vi "LabVIEW_Set Temperature.vi"(0 "PC Comms Port":refnum<visa-resource-name>="COM3", 5 "Air Temperature Setpoint (°C)":dbl=37.5 min=25.0 max=80.0 step=0.1, 11 "error in (no error)":errorcluster) -> (4 "PC Comms Port Out":refnum<visa-resource-name>="COM3", 15 "error out":errorcluster)   [LabVIEW 2010]
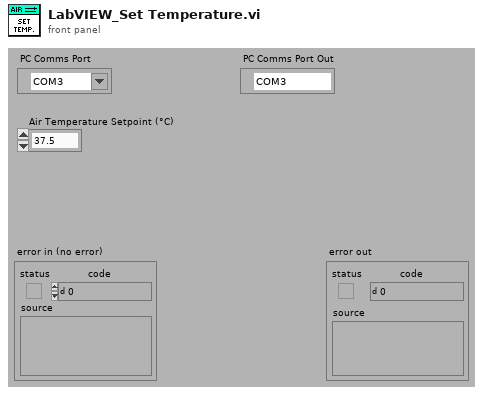
[diagram p1: front panel]
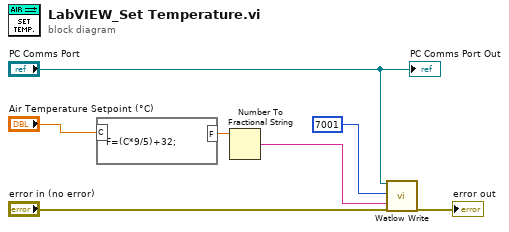
[diagram p0: block diagram]
diagram:
  n1 = formula code="F=(C*9/5)+32;"("C"="Air Temperature Setpoint (°C)") -> ("F"=w6:dbl)
  n2 = Number To Fractional String(number=w6) -> (F-format string=w5:string)  [unwired: 3 in]
  n3 = call <instrlib>:"Watlow Write.vi"("PC Comms Port"="PC Comms Port", "Parameter"=u32 7001, "Write Value"=w5, "Error In"="error in (no error)") -> ("Error Out"=→"error out":errorcluster)  [unwired: 15 in]
  "PC Comms Port Out" <- "PC Comms Port"
